vi "Main.vi"() -> ()   [LabVIEW 2013]
uses:
  <vilib>/myRIO/Instrument Drivers/Onboard IO/Encoder/vis/Smart Open.vi
  <vilib>/myRIO/Instrument Drivers/Onboard IO/Encoder/vis/Read.vi
  <vilib>/myRIO/Instrument Drivers/Onboard IO/PWM/vis/Smart Open.vi
  <vilib>/myRIO/Instrument Drivers/Onboard IO/PWM/vis/Set Duty Cycle and Frequency.vi
  <vilib>/myRIO/Instrument Drivers/Onboard IO/DIO/vis/Smart Open.vi
  <vilib>/myRIO/Instrument Drivers/Onboard IO/DIO/vis/Write.vi
  <vilib>/myRIO/Common/Instrument Driver Framework/myRIO v1.0/UART/vis/myRIO v1.0 Close UART.vi
  <vilib>/myRIO/Instrument Drivers/Onboard IO/Encoder/vis/Open.vi
  <vilib>/myRIO/Instrument Drivers/Onboard IO/PWM/vis/Open.vi
  <vilib>/myRIO/Instrument Drivers/Onboard IO/DIO/vis/Open.vi
  <vilib>/addons/control/pid/pid.llb/PID Control Input Filter (DBL).vi
  <vilib>/addons/control/pid/pid.llb/PID (DBL).vi
  <vilib>/Utility/error.llb/Error Cluster From Error Code.vi
  <vilib>/myRIO/Common/Instrument Driver Framework/Utilities/vis/FPGA Ref Manager.vi
  <vilib>/myRIO/Common/Instrument Driver Framework/myRIO v1.0/myRIO v1.0 Reset FPGA.vi
  <vilib>/myRIO/Instrument Drivers/Utilities/Utilities.lvlib
  <vilib>/addons/control/pid/NI_PID_pid.lvlib
panel:
  out "Outpur":cluster{i32[], dbl[]}[](graph)
  out "Pendulum Counter":i32
  in  "Reset Counter Pendulum":bool
  out "Pendulum Ang (deg)":dbl
  out "Numeric Control":i32
  out "Pemdulum Angle":cluster{i32[], dbl[]}[](graph)
  out "stop":bool
  in  "setpoint":dbl format="%#_13g"
  in  "PID gains":T1={"proportional gain (Kc)"=20.0, "integral time (Ti, min)"=0.0, "derivative time (Td, min)"=0.002} {"derivative time (Td, min)" format="%.3f"; "integral time (Ti, min)" format="%.3f"; "proportional gain (Kc)" format="%.3f"}
  out "Position (cm)":cluster{i32[], dbl[]}[](graph)
  out "Speed (cm/s)":dbl
  out "Distance (cm)":dbl
  in  "Frequency":dbl(slide)=500.0 scale=40.0..4000.0
  out "RPM":dbl
  out "Carriage Angle (deg)":dbl
  out "Direction":bool
  in  "Enable":bool
  out "PWM duty  [%]":dbl(slide) scale=0.0..100.0
  in  "Reset Counter":bool
  out "Carriage Counter":i32
  in  "[ESC]":bool
  # "IP-MAN DEMO #1"
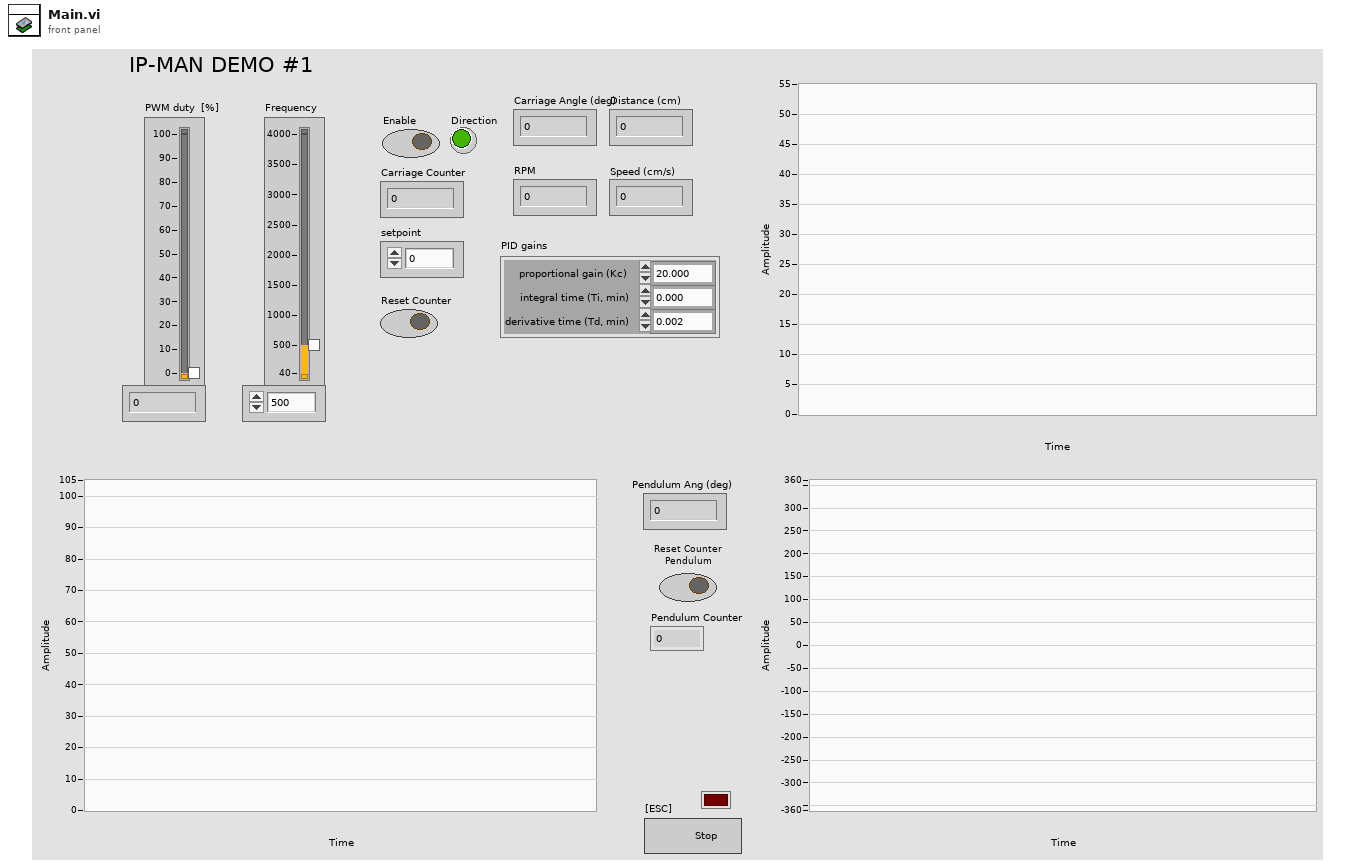
[diagram p1: front panel]
types:
  T1 = cluster{"proportional gain (Kc)":dbl, "integral time (Ti, min)":dbl, "derivative time (Td, min)":dbl}
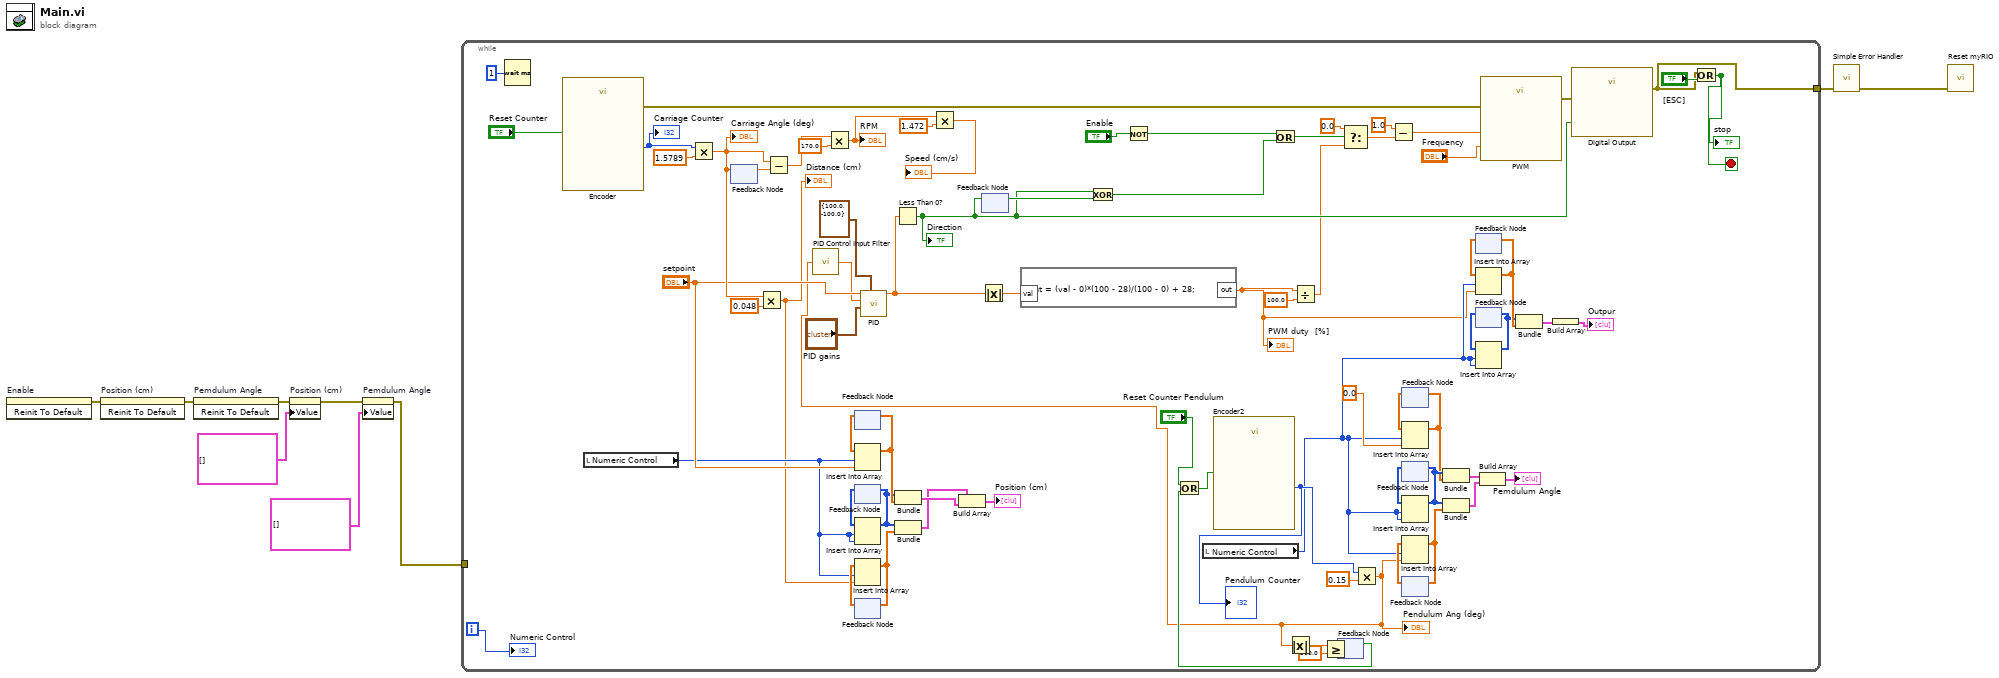
[diagram p0: block diagram]
diagram:
  n1 = invoke on="Enable" class="Bool (strict)" method="Reinit To Default"() -> (error out=w4:errorcluster)  [unwired: 3 in, 2 out]
  n2 = invoke on="Position (cm)" class="XYGraph (strict)" method="Reinit To Default"(error in=w4) -> (error out=w5:errorcluster)  [unwired: 2 in, 2 out]
  n3 = invoke on="Pemdulum Angle" class="XYGraph (strict)" method="Reinit To Default"(error in=w5) -> (error out=w3:errorcluster)  [unwired: 2 in, 2 out]
  n4 = property on="Position (cm)" class="XYGraph (strict)"(error in=w3, "Value"=cluster{i32[], dbl[]}[] [] ("Position (cm)")) -> (error out=w2:errorcluster)  [unwired: 1 in, 1 out]
  n5 = property on="Pemdulum Angle" class="XYGraph (strict)"(error in=w2, "Value"=cluster{i32[], dbl[]}[] [] ("Pemdulum Angle")) -> (error out=w1:errorcluster)  [unwired: 1 in, 1 out]
  n6 = while {
    tunnel: [w81] -> w8
    tunnel: w1 -> [_]
    i -> [w44]
    stop <- w54 stop-if-true
    n7 = Wait (ms)(milliseconds to wait=u32 1) -> ()  [unwired: 1 out]
    n8 = call "Encoder"("Reset Counter"="Reset Counter") -> ("Counter Value"=w59:i32, "error out"=w66:errorcluster)  [unwired: 23 in, 2 out]
    "Carriage Counter" <- w59
    n9 = local read "Numeric Control"() -> (w37:i32)
    n10 = Multiply(x=w59, y=1.5789) -> (x*y=w57:dbl)
    "Carriage Angle (deg)" <- w57
    n11 = feedback #1() -> (w60:dbl)  [unwired: 1 in]
    n12 = feedback-in #1(w57) -> ()
    n13 = Multiply(x=w57, y=0.048) -> (x*y=w27:dbl)
    "Distance (cm)" <- w27
    n14 = Subtract(x=w57, y=w60) -> (x-y=w75:dbl)
    n15 = Multiply(x=w75, y=170.0) -> (x*y=w63:dbl)
    "RPM" <- w63
    n16 = feedback #2() -> (w50:dbl[])  [unwired: 1 in]
    n17 = Insert Into Array(array=w50, index=w37, new element="setpoint") -> (w46:dbl[])
    n18 = feedback-in #2(w46) -> ()
    n19 = feedback #3() -> (w52:i32[])  [unwired: 1 in]
    n20 = Insert Into Array(array=w52, index=w37, new element=w37) -> (w45:i32[])
    n21 = feedback-in #3(w45) -> ()
    n22 = feedback #4() -> (w51:dbl[])  [unwired: 1 in]
    n23 = Insert Into Array(array=w51, index=w37, new element=w27) -> (w47:dbl[])
    n24 = feedback-in #4(w47) -> ()
    n25 = Bundle(w45, w46) -> (w30:cluster{i32[], dbl[]})  [unwired: 1 in]
    n26 = Bundle(w45, w47) -> (w29:cluster{i32[], dbl[]})  [unwired: 1 in]
    n27 = Multiply(x=w63, y=1.472) -> (x*y=→"Speed (cm/s)":dbl)
    n28 = Build Array(w29, w30) -> (→"Position (cm)":cluster{i32[], dbl[]}[])
    n29 = feedback #5() -> (w82:bool)  [unwired: 1 in]
    n30 = Not(x="Enable") -> (.not. x?=w78:bool)
    n31 = local read "Numeric Control"() -> (w20:i32)
    n32 = feedback #6() -> (w11:bool)  [unwired: 1 in]
    n33 = Or(x="Reset Counter Pendulum", y=w11) -> (x .or. y?=w14:bool)
    n34 = call "Encoder2"("Reset Counter"=w14) -> ("Counter Value"=w33:i32)  [unwired: 23 in, 3 out]
    "Pendulum Counter" <- w33
    n35 = Multiply(x=w33, y=0.15) -> (x*y=w10:dbl)
    "Pendulum Ang (deg)" <- w10
    n36 = call-poly <vilib>:"PID Control Input Filter.vi"("input"=w10) -> ("output"=w17:dbl)  [unwired: 4 in]
    n37 = call-poly <vilib>:"PID.vi"("output range"=cluster{"output high":dbl, "output low":dbl} {"output high"=100.0, "output low"=-100.0}, "PID gains"="PID gains", "process variable"=w17, "setpoint"="setpoint") -> ("output"=w56:dbl)  [unwired: 6 in, 1 out]
    n38 = Less Than 0?(x=w56) -> (x < 0?=w71:bool)
    "Direction" <- w71
    n39 = Absolute Value(x=w56) -> (abs(x)=w55:dbl)
    n40 = feedback-in #5(w71) -> ()
    n41 = formula code="out = (val - 0)*(100 - 28)/(100 - 0) + 28;"("val"=w55) -> ("out"=w18:dbl)
    "PWM duty  [%]" <- w18
    n42 = Exclusive Or(1:w82, 2:w71) -> (0:w80:bool)
    n43 = Or(x=w78, y=w80) -> (x .or. y?=w79:bool)
    n44 = Absolute Value(x=w10) -> (abs(x)=w16:dbl)
    n45 = Divide(x=w18, y=100.0) -> (x/y=w21:dbl)
    n46 = Greater Or Equal?(x=w16, y=360.0) -> (x >= y?=w12:bool)
    n47 = feedback-in #6(w12) -> ()
    n48 = Select(t=0.0 ("f"), s=w79, f=w21) -> (s? t:f=w70:dbl)
    n49 = Subtract(x=1.0, y=w70) -> (x-y=w69:dbl)
    n50 = feedback #7() -> (w39:dbl[])  [unwired: 1 in]
    n51 = Insert Into Array(array=w39, index=w20, new element=0.0) -> (w41:dbl[])
    n52 = feedback-in #7(w41) -> ()
    n53 = feedback #8() -> (w36:i32[])  [unwired: 1 in]
    n54 = Insert Into Array(array=w36, index=w20, new element=w20) -> (w42:i32[])
    n55 = feedback-in #8(w42) -> ()
    n56 = feedback #9() -> (w35:dbl[])  [unwired: 1 in]
    n57 = Insert Into Array(array=w35, index=w20, new element=w10) -> (w40:dbl[])
    n58 = feedback-in #9(w40) -> ()
    n59 = Bundle(w42, w41) -> (w43:cluster{i32[], dbl[]})  [unwired: 1 in]
    n60 = Bundle(w42, w40) -> (w32:cluster{i32[], dbl[]})  [unwired: 1 in]
    n61 = feedback #10() -> (w22:dbl[])  [unwired: 1 in]
    n62 = Insert Into Array(array=w22, index=w20, new element=w18) -> (w26:dbl[])
    n63 = feedback-in #10(w26) -> ()
    n64 = feedback #11() -> (w23:i32[])  [unwired: 1 in]
    n65 = Insert Into Array(array=w23, index=w20, new element=w20) -> (w25:i32[])
    n66 = feedback-in #11(w25) -> ()
    n67 = Build Array(w43, w32) -> (→"Pemdulum Angle":cluster{i32[], dbl[]}[])
    n68 = call "PWM"("Duty Cycle (0-1)"=w69, "Frequency (Hz)"="Frequency", "error in (no error)"=w66) -> ("error out"=w67:errorcluster)  [unwired: 24 in]
    n69 = Bundle(w25, w26) -> (w24:cluster{i32[], dbl[]})  [unwired: 1 in]
    n70 = Build Array(w24) -> (→"Outpur":cluster{i32[], dbl[]}[])
    n71 = call "Digital Output"("A/DIO6 (Pin 23)"=w71, "error in (no error)"=w67) -> ("error out"=w81:errorcluster)  [unwired: 25 in]
    n72 = Or(x=w81, y="[ESC]") -> (x .or. y?=w54:bool)
    "stop" <- w54
    "Numeric Control" <- w44
  }
  n73 = call <vilib>:"Simple Error Handler.vi"("error in (no error)"=w8) -> ("error out"=w9:errorcluster)  [unwired: 4 in, 4 out]
  n74 = call <vilib>:"Reset myRIO.vi"("error in (no error)"=w9) -> ()  [unwired: 10 in, 1 out]
